vi "LLNodeProbe.vi"(11 "LLNode":refnum<class "LLNode.lvclass">) -> (2 "Value String":string, 3 "Boolean":bool)   [LabVIEW 2009, in "LLNode.lvclass"]
uses:
  LLNode.lvclass
panel:
  in  "Linked List Nodes":i32(listbox)
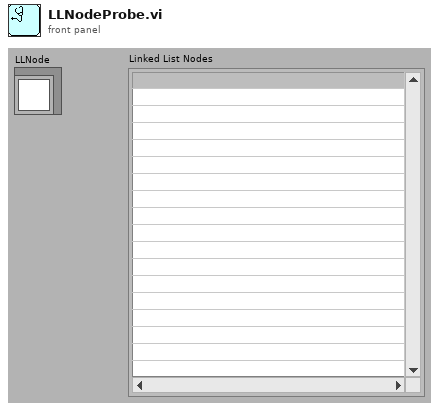
[diagram p1: front panel]
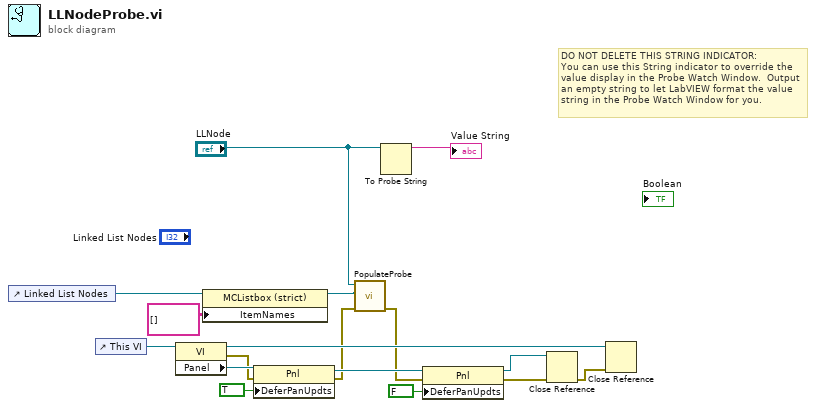
[diagram p0: block diagram]
diagram:
  # "DO NOT DELETE THIS STRING INDICATOR: \nYou can use this String indicator to override the value display in the Probe Watch Window.  Output an empty string to let LabVIEW format the value string in the Probe Watch Window for you."
  n1 = control-ref of="Linked List Nodes"() -> (w1:refnum<vi>)
  n2 = control-ref of="This VI"() -> (w16:refnum<vi>)
  n3 = property class="VI"(reference=w16) -> (reference out=w7:refnum<vi>, error out=w14:errorcluster, "Panel"=w15:refnum<vi>)  [unwired: 1 in]
  n4 = property class="MCListbox (strict)"(reference=w1, "ItemNames"=string[][] [] ("Item Names")) -> (reference out=w4:refnum<vi>)  [unwired: 1 in, 1 out]
  n5 = property class="Pnl"(reference=w15, error in=w14, "DeferPanUpdts"=TRUE ("Defer Panel Updates")) -> (reference out=w12:refnum<vi>, error out=w3:errorcluster)
  n6 = call-dynamic "PopulateProbe.vi"("error in (no error)"=w3, "Multicolumn Listbox in"=w4, "LLNode in"="LLNode") -> ("error out"=w2:errorcluster)  [unwired: 6 in, 2 out]
  n7 = To Probe String(7:"LLNode") -> (3:→"Value String":string)  [unwired: 2 in, 1 out]
  n8 = property class="Pnl"(reference=w12, error in=w2, "DeferPanUpdts"=FALSE ("Defer Panel Updates")) -> (reference out=w9:refnum<vi>, error out=w10:errorcluster)
  n9 = Close Reference(reference=w9, error in (no error)=w10) -> (error out=w8:errorcluster)
  n10 = Close Reference(reference=w7, error in (no error)=w8) -> ()  [unwired: 1 out]
